vi "sub_replace_self.vi"(0 "path to generate code ability":path, 1 "Diagram":T6, 2 "XRef":T11, 3 "State In":T1 {"BlockNodeState"."Draw Style" items=["FunctionBlock", "ExpressVI", "Variable", "Elemental I/O", "32x32 Icon", "FunctionBlockCompact"]; "BlockNodeState"."Terminal Data"."Terminal Flags" format="%.0b"}, 4 "Terms":T7) -> (16 "Generated Code?":T12)   [LabVIEW 2018]
uses:
  <vilib>/XNodeSupport/XNodeBool.ctl
  <vilib>/XNodeSupport/XNodeXNodeRef.ctl
  <vilib>/XNodeSupport/XNodeTermIDPairs.ctl
  <vilib>/XNodeSupport/XNodeTermIDPair.ctl
  <vilib>/XNodeSupport/XNodeTermRef.ctl
  <vilib>/XNodeSupport/XNodeString.ctl
  <vilib>/XNodeSupport/XNodeTopLevelDiagramRef.ctl
  State.ctl
  <vilib>/BlockNodeSupport/BlockNodeState.ctl
  <vilib>/BlockNodeSupport/TerminalData.ctl
  <vilib>/picture/picture.llb/imagedata.ctl
  command_spec.ctl
  <vilib>/Utility/miscctls.llb/LVPointTypeDef.ctl
  <vilib>/XNodeSupport/NI_XNodeSupport.lvlib
  N9010A_SCPI Node.xnode
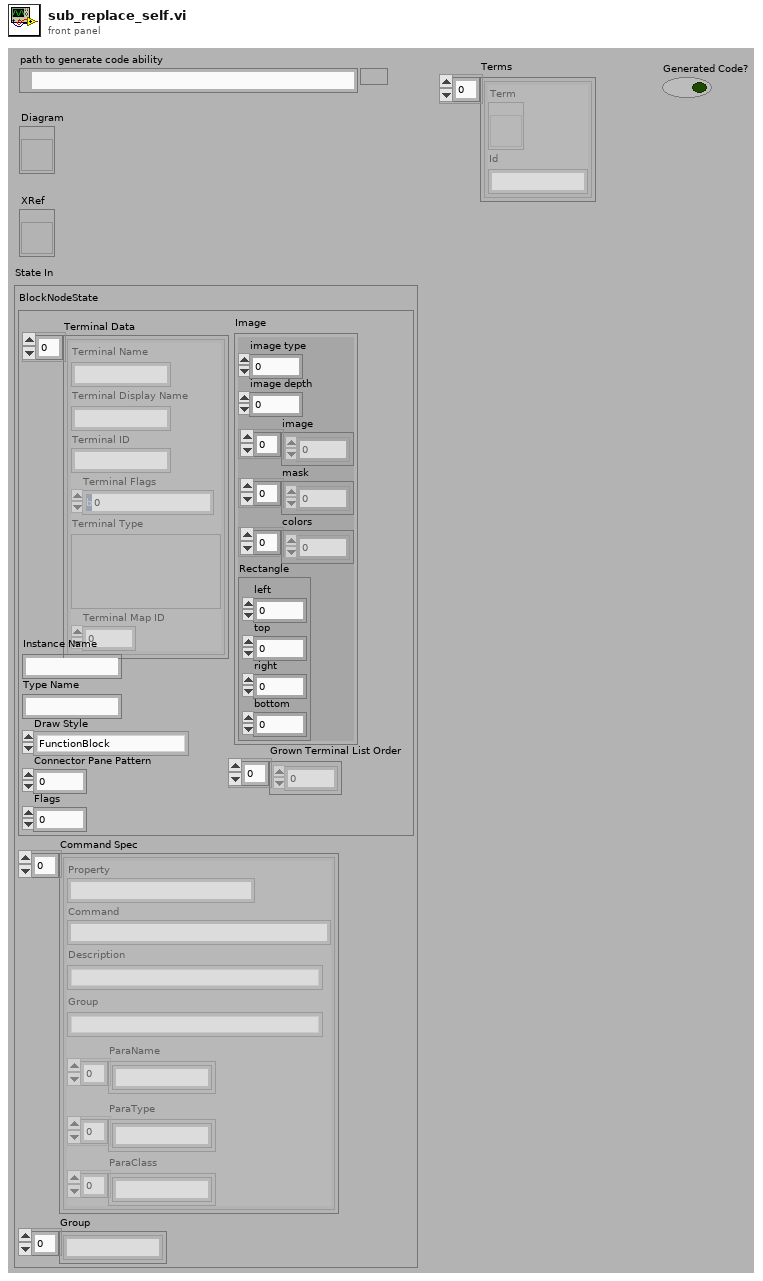
[diagram p1: front panel]
types:
  T1 = typedef "N9010A_SCPI Node.xnode/State.ctl" = cluster{"BlockNodeState":T2, "Command Spec":T5, "Group":string[]}
  T2 = typedef "BlockNodeState.ctl" = cluster{"Terminal Data":T3[], "Instance Name":string, "Type Name":string, "Draw Style":i32, "Connector Pane Pattern":i32, "Flags":i32, "Grown Terminal List Order":i32[], "Image":T4}
  T3 = typedef "TerminalData.ctl" = cluster{"Terminal Name":string, "Terminal Display Name":string, "Terminal ID":string, "Terminal Flags":i32, "Terminal Type":variant, "Terminal Map ID":i32}
  T4 = typedef "imagedata.ctl" = cluster{"image type":i32, "image depth":i32, "image":u8[], "mask":u8[], "colors":u32[], "Rectangle":cluster{"left":i16, "top":i16, "right":i16, "bottom":i16}}
  T5 = typedef "command_spec.ctl" = cluster{"Property":string, "Command":string, "Description":string, "Group":string, "ParaName":string[], "ParaType":string[], "ParaClass":string[]}[]
  T6 = typedef "NI_XNodeSupport.lvlib/XNodeTopLevelDiagramRef.ctl" = refnum<vi>
  T7 = typedef "NI_XNodeSupport.lvlib/XNodeTermIDPairs.ctl" = T8[]
  T8 = typedef "NI_XNodeSupport.lvlib/XNodeTermIDPair.ctl" = cluster{"Term":T9, "Id":T10}
  T9 = typedef "NI_XNodeSupport.lvlib/XNodeTermRef.ctl" = refnum<vi>
  T10 = typedef "NI_XNodeSupport.lvlib/XNodeString.ctl" = string
  T11 = typedef "NI_XNodeSupport.lvlib/XNodeXNodeRef.ctl" = refnum<vi>
  T12 = typedef "NI_XNodeSupport.lvlib/XNodeBool.ctl" = bool
  T13 = typedef "LVPointTypeDef.ctl" = cluster{"Horizontal":i16, "Vertical":i16}
  T14 = typedef "LVRectTypeDef.ctl" = cluster{"Left":i16, "Top":i16, "Right":i16, "Bottom":i16}
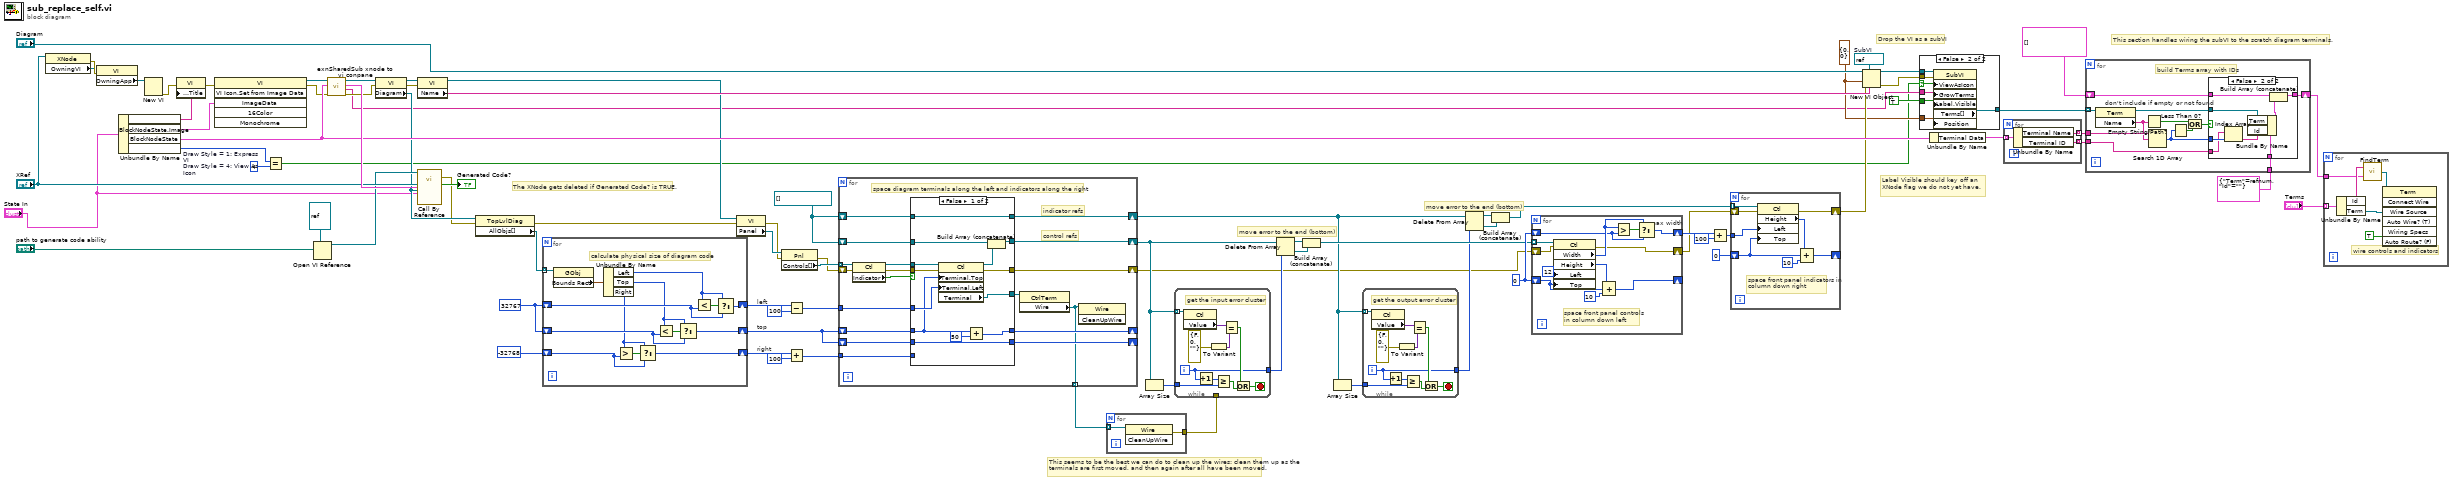
[diagram p0: block diagram]
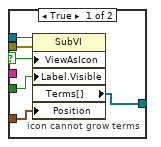
[diagram p2: hidden frame]
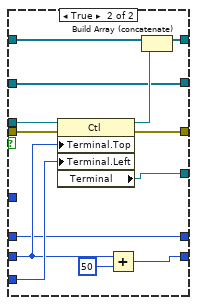
[diagram p3: hidden frame]
diagram:
  w30 = 0 ("Position:Left")
  w31 = refnum<vi>[] []
  w47 = i16 32767 ("left")
  w66 = refnum<vi> refnum  # SubVI
  w7 = T13 {"Horizontal"=0, "Vertical"=0} ("relative position/next to refnum")
  w54 = 4  # Draw Style = 1: Express VI Draw Style = 4: View As Icon
  # "The XNode gets deleted if Generated Code? is TRUE."
  # "Label Visible should key off an XNode flag we do not yet have."
  # "This seems to be the best we can do to clean up the wires: clean them up as the terminals are first moved, and then again after all have been moved."
  # "move error to the end (bottom)"
  # "move error to the end (bottom)"
  # "right"
  # "top"
  # "left"
  # "Drop the VI as a subVI"
  # "This section handles wiring the subVI to the scratch diagram terminals."
  n1 = property class="XNode"(reference="XRef") -> (error out=w62:errorcluster, "OwningVI"=w61:refnum<vi>)  [unwired: 1 in, 1 out]
  n2 = property class="VI"(reference=w61, error in=w62) -> ("OwningApp"=w63:refnum<vi>)  [unwired: 2 out]
  n3 = Unbundle By Name("State In") -> ("BlockNodeState.Type Name"=w53:string, "BlockNodeState.Image"=w52:T4, "BlockNodeState"=w69:T2, "BlockNodeState.Draw Style"=w5:i32)
  n4 = New VI(11:w63) -> (0:w56:errorcluster)  [unwired: 1 in, 6 out]
  n5 = property class="VI"(error in=w56, "Front Panel.Title"=w53) -> (error out=w51:errorcluster)  [unwired: 1 in, 1 out]
  n6 = invoke class="VI" method="VI Icon.Set from Image Data"(error in=w51, "ImageData"=w52) -> (reference out=w1:refnum<vi>, error out=w55:errorcluster)  [unwired: 4 in, 4 out]
  n7 = Equal?(x=w5, y=w54) -> (x = y?=w3:bool)
  n8 = Open VI Reference(type specifier VI Refnum (for type only)=refnum<vi> refnum, vi path="path to generate code ability") -> (vi reference=w78:refnum<vi>)  [unwired: 1 in, 4 out]
  n9 = call <vilib>:"exnSharedSub xnode to vi conpane.vi"("error in (no error)"=w55, "BlockNodeState"=w69, "VI Refnum"=w1) -> ("error out"=w58:errorcluster, "GrownTerms"=w6:string[], "Terms"=w81:T7, "VI Refnum out"=w57:refnum<vi>)  [unwired: 5 out]
  n10 = property class="VI"(reference=w57, error in=w58) -> (reference out=w60:refnum<vi>, error out=w59:errorcluster, "Diagram"=w49:refnum<vi>)
  n11 = property class="VI"(reference=w60, error in=w59) -> (reference out=w36:refnum<vi>, "Name"=w65:string)  [unwired: 1 out]
  n12 = call-by-ref "?"(reference=w78, "XRef"="XRef", "Terms"=w81, "Diagram"=w49, "State In"="State In") -> (error out=w38:errorcluster, "Generated Code?"=→"Generated Code?":T12)  [unwired: 14 in, 3 out]
  n13 = property class="TopLvlDiag"(reference=w49, error in=w38) -> (error out=w37:errorcluster, "AllObjs[]"=w48:refnum<vi>[])  [unwired: 1 out]
  n14 = for {
    tunnel: w48 -> [w95] mode=indexing
    shift-right: [w91] -> w45
    shift-left: w47 -> [w89]
    shift-right: [w92] -> w39
    shift-left: w47 -> [w86]
    shift-right: [w93] -> w41
    shift-left: i16 -32768 ("left") -> [w82]
    # "calculate physical size of diagram code"
    n15 = property class="GObj"(reference=w95) -> ("Bounds Rect"=w94:T14)  [unwired: 1 in, 2 out]
    n16 = Unbundle By Name(w94) -> ("Left"=w83:i16, "Top"=w84:i16, "Right"=w85:i16)
    n17 = Greater?(x=w85, y=w82) -> (0:w87:bool)
    n18 = Select(t=w85, s=w87, f=w82) -> (s? t:f=w93:i16)
    n19 = Less?(x=w84, y=w86) -> (x < y?=w88:bool)
    n20 = Select(t=w84, s=w88, f=w86) -> (s? t:f=w92:i16)
    n21 = Less?(x=w83, y=w89) -> (x < y?=w90:bool)
    n22 = Select(t=w83, s=w90, f=w89) -> (s? t:f=w91:i16)
  }
  n23 = property class="VI"(reference=w36, error in=w37) -> (error out=w33:errorcluster, "Panel"=w35:refnum<vi>)  [unwired: 1 out]
  n24 = property class="Pnl"(reference=w35, error in=w33) -> (error out=w32:errorcluster, "Controls[]"=w34:refnum<vi>[])  [unwired: 1 out]
  n25 = Subtract(x=w45, y=i16 100) -> (x-y=w44:i16)
  n26 = Add(x=w41, y=i16 100) -> (x+y=w40:i16)
  n27 = for {
    tunnel: w44 -> [w108]
    tunnel: w40 -> [w113]
    shift-right: [w109] -> _
    shift-left: w39 -> [w110]
    shift-right: [w111] -> _
    shift-left: w39 -> [w112]
    tunnel: w34 -> [w105] mode=indexing
    shift-right: [w103] -> w9
    shift-left: w32 -> [w102]
    shift-right: [w99] -> w19
    shift-left: w31 -> [w100]
    shift-right: [w97] -> w12
    shift-left: w31 -> [w98]
    tunnel: [w96] -> w11 mode=indexing
    # "indicator refs"
    # "control refs"
    # "space diagram terminals along the left and indicators along the right"
    n28 = property class="Ctl"(reference=w105, error in=w102) -> (reference out=w107:refnum<vi>, error out=w104:errorcluster, "Indicator"=w106:bool)
    n29 = case shown="False" w106 {
      tunnel: w107 -> [w126 w139]
      tunnel: w113 -> [_ w138]
      tunnel: w112 -> [w122 w136]
      tunnel: [w122 w135] -> w111
      tunnel: w110 -> [w119 w134]
      tunnel: [w123 w134] -> w109
      tunnel: w108 -> [w124 _]
      tunnel: w104 -> [w120 w133]
      tunnel: [w121 w132] -> w103
      tunnel: [w118 w131] -> w101
      tunnel: w100 -> [w116 w129]
      tunnel: [w115 w129] -> w99
      tunnel: w98 -> [w114 w128]
      tunnel: [w114 w127] -> w97
      frame False {
        n30 = property class="Ctl"(reference=w126, error in=w120, "Terminal.Top"=w119, "Terminal.Left"=w124) -> (reference out=w117:refnum<vi>, error out=w121:errorcluster, "Terminal"=w118:refnum<vi>)
        n31 = Add(x=w119, y=i16 50) -> (x+y=w123:i16)
        n32 = Build Array (concatenate)(w116, w117) -> (w115:refnum<vi>[])
      }
      frame True {
        n33 = property class="Ctl"(reference=w139, error in=w133, "Terminal.Top"=w136, "Terminal.Left"=w138) -> (reference out=w130:refnum<vi>, error out=w132:errorcluster, "Terminal"=w131:refnum<vi>)
        n34 = Add(x=w136, y=i16 50) -> (x+y=w135:i16)
        n35 = Build Array (concatenate)(w128, w130) -> (w127:refnum<vi>[])
      }
    }
    n36 = property class="CtrlTerm"(reference=w101) -> ("Wire"=w96:refnum<vi>)  [unwired: 1 in, 2 out]
    n37 = invoke class="Wire" method="CleanUpWire"(reference=w96) -> ()  [unwired: 2 in, 3 out]
  }
  n38 = for {
    tunnel: w11 -> [w141] mode=indexing
    tunnel: [w140] -> w10
    n39 = invoke class="Wire" method="CleanUpWire"(reference=w141) -> (error out=w140:errorcluster)  [unwired: 2 in, 2 out]
  }
  n40 = Array Size(array=w19) -> (size(s)=w23:i32)
  n41 = while {
    tunnel: w19 -> [w151] mode=indexing
    tunnel: w23 -> [w146]
    tunnel: [w142] -> w22
    tunnel: w10 -> [_]
    i -> [w142]
    stop <- w144 stop-if-true
    # "get the input error cluster"
    n42 = property class="Ctl"(reference=w151) -> ("Value"=w150:variant)  [unwired: 1 in, 2 out]
    n43 = Increment(x=w142) -> (x+1=w143:i32)
    n44 = To Variant(anything=errorcluster {"status"=FALSE, "code"=0, "source"=""} ("error in (no error)")) -> (Variant=w148:variant)
    n45 = Greater Or Equal?(x=w143, y=w146) -> (x >= y?=w145:bool)
    n46 = Equal?(x=w150, y=w148) -> (x = y?=w147:bool)
    n47 = Or(x=w147, y=w145) -> (x .or. y?=w144:bool)
  }
  n48 = Delete From Array(array=w19, index=w22) -> (deleted portion=w20:refnum<vi>, array with subset deleted=w21:refnum<vi>[])  [unwired: 1 in]
  n49 = Build Array (concatenate)(w21, w20) -> (w18:refnum<vi>[])
  n50 = Array Size(array=w12) -> (size(s)=w17:i32)
  n51 = while {
    tunnel: w12 -> [w161] mode=indexing
    tunnel: w17 -> [w156]
    tunnel: [w153] -> w14
    i -> [w153]
    stop <- w154 stop-if-true
    # "get the output error cluster"
    n52 = property class="Ctl"(reference=w161) -> ("Value"=w160:variant)  [unwired: 1 in, 2 out]
    n53 = Increment(x=w153) -> (x+1=w152:i32)
    n54 = To Variant(anything=errorcluster {"status"=FALSE, "code"=0, "source"=""} ("error in (no error)")) -> (Variant=w158:variant)
    n55 = Greater Or Equal?(x=w152, y=w156) -> (x >= y?=w155:bool)
    n56 = Equal?(x=w160, y=w158) -> (x = y?=w157:bool)
    n57 = Or(x=w157, y=w155) -> (x .or. y?=w154:bool)
  }
  n58 = Delete From Array(array=w12, index=w14) -> (deleted portion=w16:refnum<vi>, array with subset deleted=w15:refnum<vi>[])  [unwired: 1 in]
  n59 = Build Array (concatenate)(w15, w16) -> (w13:refnum<vi>[])
  n60 = for {
    tunnel: w18 -> [w173] mode=indexing
    shift-right: [w168] -> _
    shift-left: w30 -> [w170]
    shift-right: [w164] -> w28
    shift-left: w30 -> [w165]
    shift-right: [w162] -> w26
    shift-left: w9 -> [w163]
    # "space front panel controls in column down left"
    # "max width"
    n61 = property class="Ctl"(reference=w173, error in=w163, "Left"=12 ("Position:Left"), "Top"=w170) -> (error out=w162:errorcluster, "Width"=w166:u32, "Height"=w171:u32)  [unwired: 1 out]
    n62 = Compound Arithmetic op=ADD(w171, w170, 10 ("value")) -> (w168:u32)
    n63 = Greater?(x=w166, y=w165) -> (0:w167:bool)
    n64 = Select(t=w166, s=w167, f=w165) -> (s? t:f=w164:u32)
  }
  n65 = Add(x=w28, y=u32 100) -> (x+y=w27:u32)
  n66 = for {
    tunnel: w13 -> [w181] mode=indexing
    tunnel: w27 -> [w180]
    shift-right: [w178] -> w24
    shift-left: w26 -> [w179]
    shift-right: [w174] -> _
    shift-left: 0 ("Position:Left") -> [w175]
    # "space front panel indicators in column down right"
    n67 = property class="Ctl"(reference=w181, error in=w179, "Left"=w180, "Top"=w175) -> (error out=w178:errorcluster, "Height"=w176:u32)  [unwired: 1 out]
    n68 = Compound Arithmetic op=ADD(w176, w175, 10 ("value")) -> (w174:u32)
  }
  n69 = New VI Object(vi object class=w66, owner refnum="Diagram", position/next to=w7, 6:w65, 8:w24) -> (object refnum=w67:refnum<vi>, 0:w4:errorcluster)  [unwired: 3 out]
  n70 = case shown="False" w3 {
    selector: w3 -> [w182 w188]
    tunnel: [w187 w194] -> w71
    tunnel: TRUE ("Label.Visible") -> [w186 w193]
    tunnel: w67 -> [w185 w192]
    tunnel: w7 -> [w184 w191]
    tunnel: w6 -> [_ w190]
    tunnel: w4 -> [w183 w189]
    frame True {
      # "icon cannot grow terms"
      n71 = property class="SubVI"(reference=w185, error in=w183, "ViewAsIcon"=w182, "Label.Visible"=w186, "Position"=w184) -> ("Terms[]"=w187:refnum<vi>[])  [unwired: 2 out]
    }
    frame False {
      n72 = property class="SubVI"(reference=w192, error in=w189, "ViewAsIcon"=w188, "GrowTerms"=w190, "Label.Visible"=w193, "Position"=w191) -> ("Terms[]"=w194:refnum<vi>[])  [unwired: 2 out]
    }
  }
  n73 = Unbundle By Name(w69) -> ("Terminal Data"=w70:T3[])
  n74 = for {
    tunnel: w70 -> [w197] mode=indexing
    tunnel: [w196] -> w72 mode=indexing
    tunnel: [w195] -> w73 mode=indexing
    n75 = Unbundle By Name(w197) -> ("Terminal Name"=w196:string, "Terminal ID"=w195:string)
  }
  n76 = for {
    tunnel: w71 -> [w209] mode=indexing
    tunnel: w72 -> [w208]
    tunnel: w73 -> [w199]
    tunnel: T8 {"Term"=refnum, "Id"=""} ("Code Gen Term") -> [w206]
    shift-right: [w204] -> w76
    shift-left: T8[] [] -> [w205]
    # "don't include if empty or not found"
    # "build Terms array with IDs"
    n77 = property class="Term"(reference=w209) -> (reference out=w207:refnum<vi>, "Name"=w198:string)  [unwired: 1 in, 1 out]
    n78 = Empty String/Path?(string/path=w198) -> (empty?=w203:bool)
    n79 = Search 1D Array(1D array=w208, element=w198) -> (index of element=w202:i32)  [unwired: 1 out]
    n80 = Less Than 0?(x=w202) -> (x < 0?=w200:bool)
    n81 = Or(x=w203, y=w200) -> (x .or. y?=w201:bool)
    n82 = case shown="False" w201 {
      tunnel: w207 -> [_ w218]
      tunnel: w206 -> [_ w215]
      tunnel: w205 -> [w210 w214]
      tunnel: [w210 w213] -> w204
      tunnel: w202 -> [_ w212]
      tunnel: w199 -> [_ w211]
      frame True {
      }
      frame False {
        n83 = Index Array(array=w211, index=w212) -> (element=w217:string)
        n84 = Bundle By Name(cluster=w215, "Term"=w218, "Id"=w217) -> (w216:T8)
        n85 = Build Array (concatenate)(w214, w216) -> (w213:T8[])
      }
    }
  }
  n86 = for {
    tunnel: "Terms" -> [w223] mode=indexing
    tunnel: w76 -> [w220]
    # "wire controls and indicators"
    n87 = Unbundle By Name(w223) -> ("Id"=w221:T10, "Term"=w222:T9)
    n88 = call <vilib>:"FindTerm.vi"("Terms"=w220, "String"=w221) -> ("Term"=w219:refnum<vi>)
    n89 = invoke class="Term" method="Connect Wire"(reference=w219, "Wire Source"=w222, "Auto Route? (F)"=TRUE) -> ()  [unwired: 4 in, 7 out]
  }
